vi "GetController.vi"(8 "error in (no error)":errorcluster, 11 "VIEW in":refnum<class "VIEW.lvclass">) -> (0 "error out":errorcluster, 2 "CONTROLLER":refnum<class "CONTROLLER.lvclass">, 3 "VIEW out":refnum<class "VIEW.lvclass">)   [LabVIEW 2013, in "VIEW.lvclass"]
uses:
  VIEW.lvclass
  Controller/base/CONTROLLER.lvclass
  VIEW.lvclass/VIEW.ctl
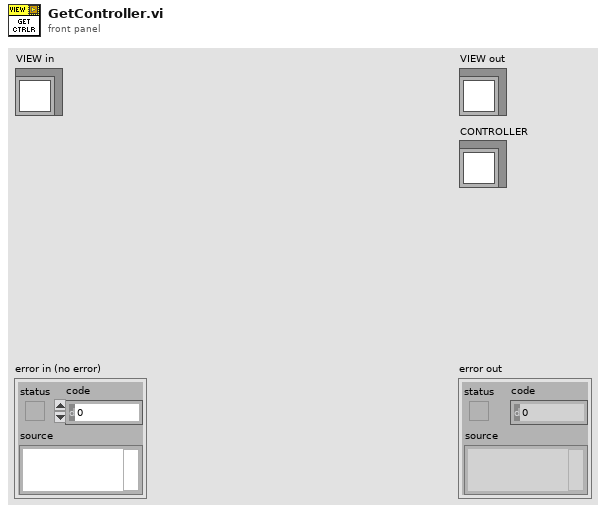
[diagram p1: front panel]
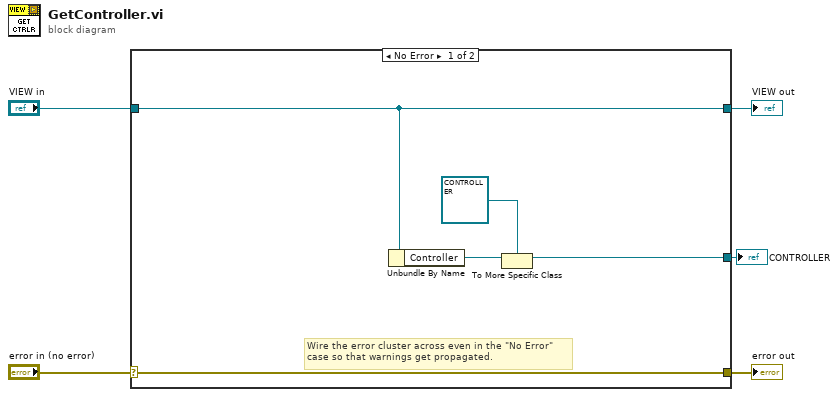
[diagram p0: block diagram]
diagram:
  n1 = case shown="No Error" "error in (no error)" {
    selector: "error in (no error)" -> [w10 w12]
    tunnel: [w10 w12] -> w4
    tunnel: [w9 w11] -> w2
    tunnel: "VIEW in" -> [w9 w11]
    tunnel: [w6 _] -> w1
    frame No Error {
      # "Wire the error cluster across even in the \"No Error\"\ncase so that warnings get propagated."
      n2 = Unbundle By Name(w9) -> ("Controller"=w8:refnum<class>)
      n3 = To More Specific Class(target class=refnum<class "CONTROLLER.lvclass"> refnum ("CONTROLLER.lvclass"), reference=w8) -> (specific class reference=w6:refnum<class "CONTROLLER.lvclass">)  [unwired: 1 in, 1 out]
    }
    frame Error {
    }
  }
  "error out" <- w4
  "VIEW out" <- w2
  "CONTROLLER" <- w1
